vi "PS2521G_SetVoltagevi.vi"(5 "GPIB Bus":i32 min=0 max=5, 6 "Channel":i16=8 max=31, 8 "error in":errorcluster, 9 "CURRENT (A)":string=".8", 10 "VOLTS":string="0", 11 "GPIB Address":i16=8 max=31) -> (0 "error out":errorcluster)   [LabVIEW 2023]
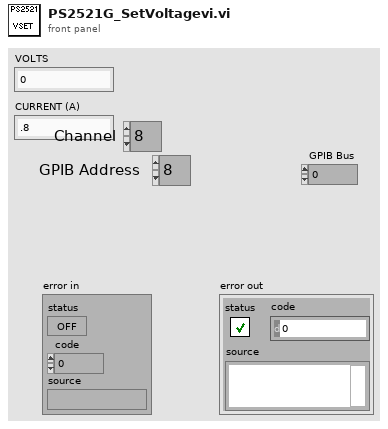
[diagram p1: front panel]
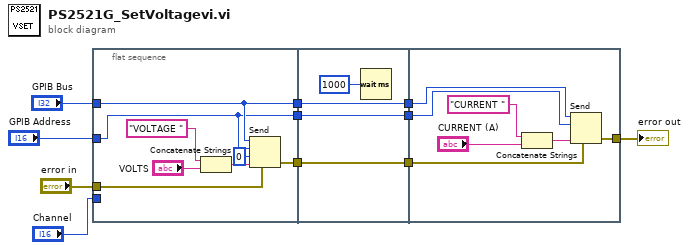
[diagram p0: block diagram]
diagram:
  n1 = flat-sequence {
    tunnel: [w15] -> w7
    tunnel: [w14] -> w5
    tunnel: [w13] -> w3
    tunnel: "GPIB Address" -> [w13]
    tunnel: "GPIB Bus" -> [w14]
    tunnel: "error in" -> [w19]
    tunnel: "Channel" -> [_]
    tunnel: w7 -> [w23]
    tunnel: [w23] -> w6
    tunnel: w5 -> [w22]
    tunnel: [w22] -> w4
    tunnel: w3 -> [w21]
    tunnel: [w21] -> w2
    tunnel: [w27] -> w8
    tunnel: w6 -> [w28]
    tunnel: w4 -> [w30]
    tunnel: w2 -> [w29]
    frame #0 {
      n2 = Concatenate Strings("VOLTAGE " ("string"), "VOLTS") -> (w18:string)
      n3 = Send(0:w14, 2:w13, 3:i16 0 ("mode"), 4:w19, 5:w18) -> (8:w15:errorcluster)  [unwired: 2 out]
    }
    frame #1 {
      n4 = Wait (ms)(milliseconds to wait=u32 1000) -> ()  [unwired: 1 out]
    }
    frame #2 {
      n5 = Concatenate Strings("CURRENT " ("string"), "CURRENT (A)") -> (w24:string)
      n6 = Send(0:w30, 2:w29, 4:w28, 5:w24) -> (8:w27:errorcluster)  [unwired: 1 in, 2 out]
    }
  }
  "error out" <- w8
